vi "Countdown.vi"() -> ()   [LabVIEW 2021]
panel:
  out "COUNTDOWN":i32
  in  "stop":bool
  in  "OK Button":bool
  # "Trigger"
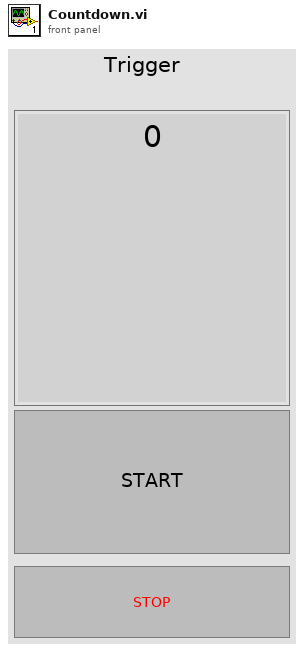
[diagram p1: front panel]
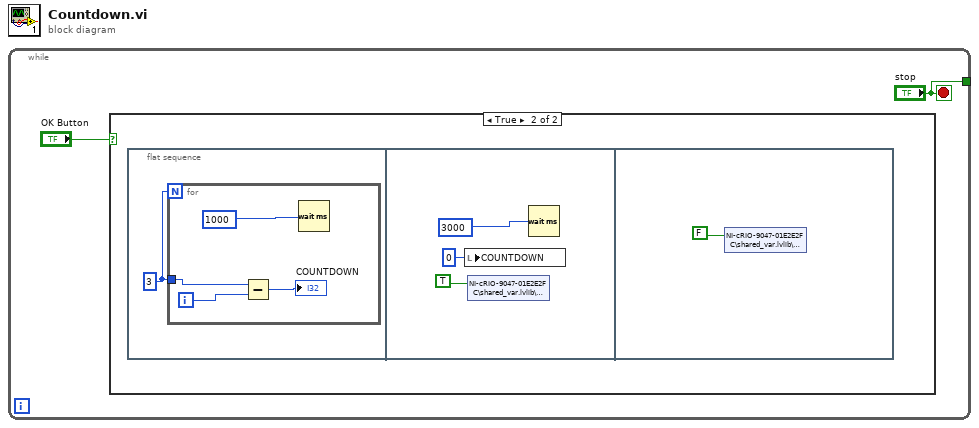
[diagram p0: block diagram]
diagram:
  n1 = while {
    tunnel: ["stop"] -> _
    stop <- "stop" stop-if-true
    n2 = case shown="True" "OK Button" {
      frame False {
      }
      frame True {
        n3 = flat-sequence {
          frame #0 {
            w3 = 3 ("y")
            n4 = for {
              N: w3 -> [_]
              tunnel: w3 -> [w4]
              i -> [w7]
              n5 = Subtract(x=w4, y=w7) -> (x-y=→"COUNTDOWN":i32)
              n6 = Wait (ms)(milliseconds to wait=u32 1000) -> ()  [unwired: 1 out]
            }
          }
          frame #1 {
            n7 = local write "COUNTDOWN"(0 ("COUNTDOWN")) -> ()
            n8 = shared-variable "NI-cRIO-9047-01E2E2FC\\shared_var.lvlib\\Trigger"(TRUE ("Trigger")) -> ()  [unwired: 1 in, 1 out]
            n9 = Wait (ms)(milliseconds to wait=u32 3000) -> ()  [unwired: 1 out]
          }
          frame #2 {
            n10 = shared-variable "NI-cRIO-9047-01E2E2FC\\shared_var.lvlib\\Trigger"(FALSE ("Trigger")) -> ()  [unwired: 1 in, 1 out]
          }
        }
      }
    }
  }
